vi "古田户外一体站流程平行样自动启动.vi"(9 "参数":T1={"是否启用仪器"=FALSE, "CODMn"={"启动测量模式"={"测量模式"=enum."水样测量"}, "确定按钮"=TRUE}, "启动模块"={"氨氮1"=FALSE, "总磷1"=FALSE, " COD1"=FALSE}, "常规启动"=FALSE, "直接启动"=FALSE}) -> ()   [LabVIEW 2016, in "质控单元.lvlib"]
uses:
  PLC/PLC.lvlib
panel:
  out "COD平行样测完标志":bool
  out "氨氮总磷平行样测完标志":bool
  out "枚举 2":enum16{"初始化", "采配水启动", "等待", "配水", "排水", "结束"}(ring)
  out "枚举":enum16{"初始化", "采配水启动", "等待", "配水", "排水", "结束"}(ring)
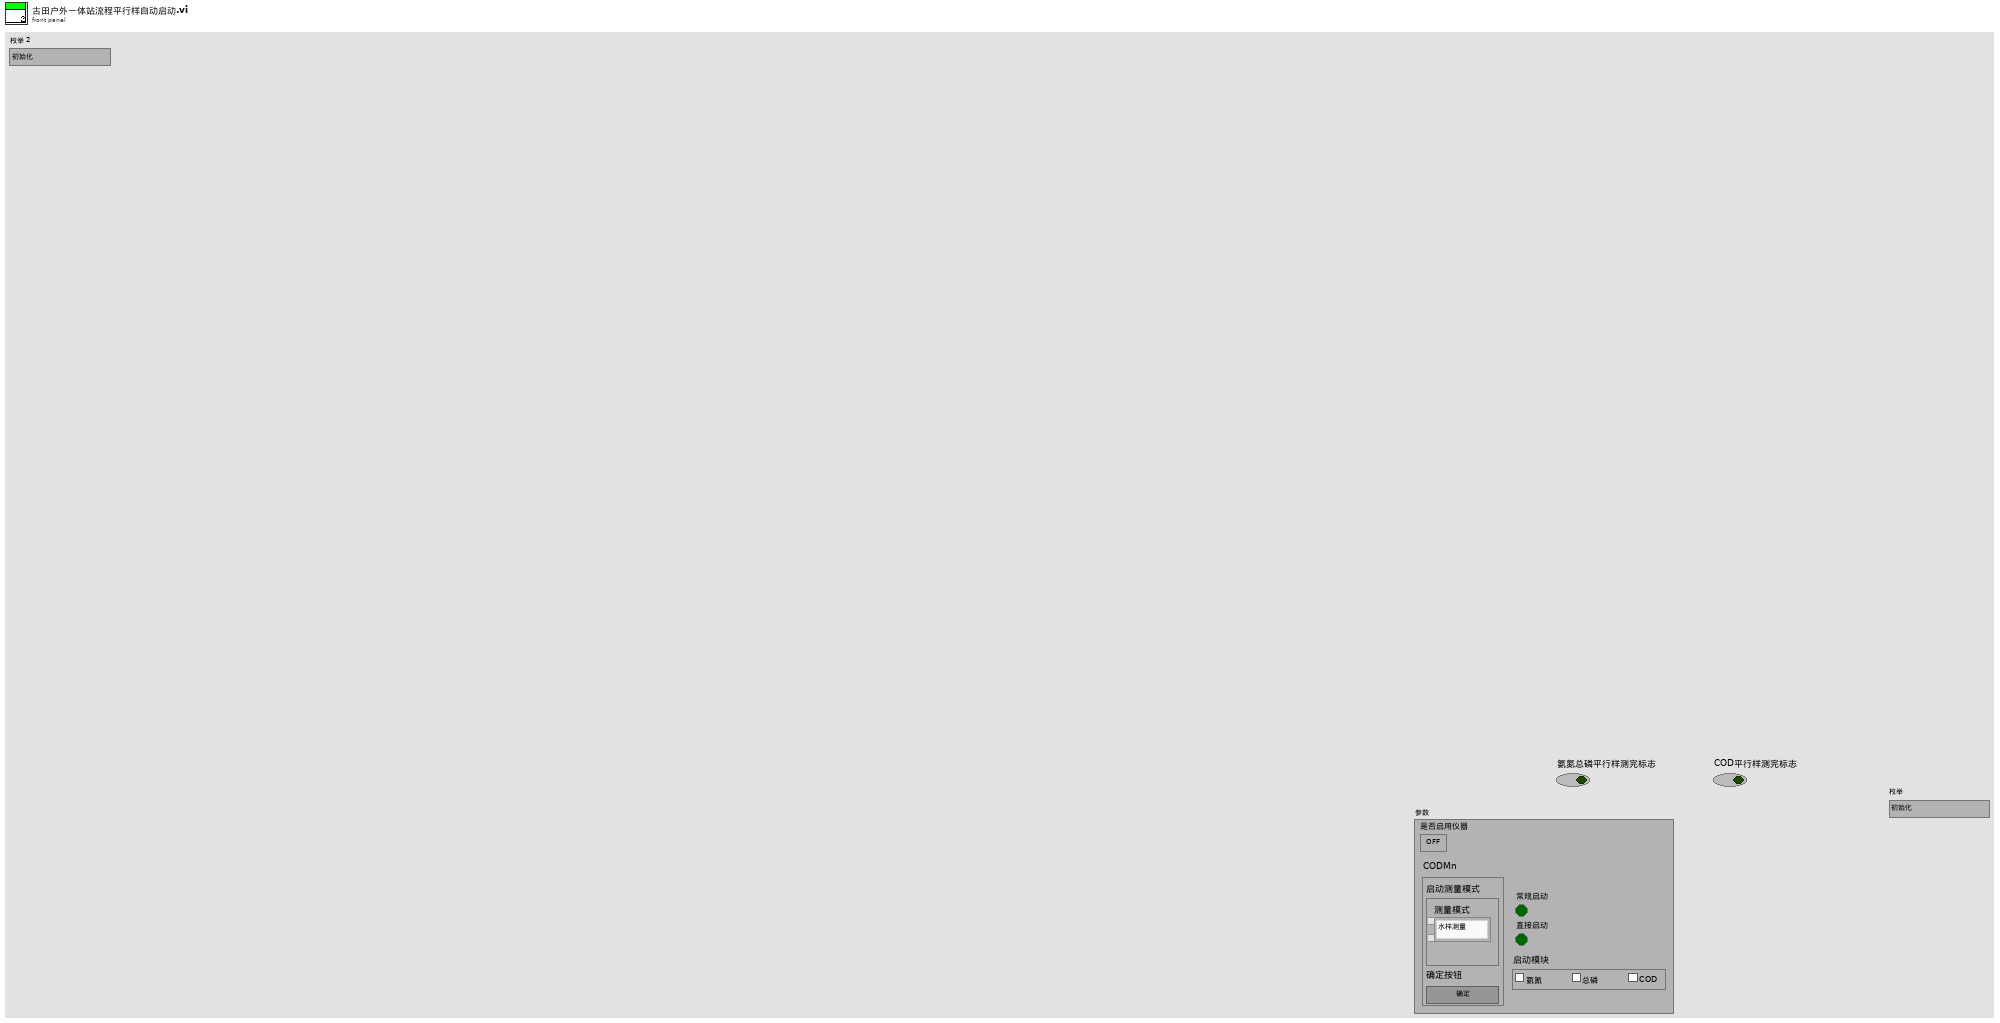
[diagram p1: front panel]
types:
  T1 = cluster{"是否启用仪器":bool, "CODMn":cluster{"启动测量模式":cluster{"测量模式":enum16{"水样测量", "标样核查", "加标回收", "平行样", "校零", "校标"}}, "确定按钮":bool}, "启动模块":cluster{"氨氮1":bool, "总磷1":bool, " COD1":bool}, "常规启动":bool, "直接启动":bool}
  T2 = cluster{"命令":string, cluster{"starting address":u16, "holding register value":u16}}
  T3 = cluster{"R0":i16, "R1":i16, "R2":i16, "R3":i16, "R4":i16, "R5":i16, "R6":i16, "R7":i16, "R8":i16, "R9":i16, "R10":i16, "R11":i16, "R12":i16, "R13":i16, "R14":i16, "R15":i16, "R16":i16, "R17":i16, "R18":i16, "R19":i16}
  T4 = enum32{"Bad", "Idle", "Run top level", "Running"}
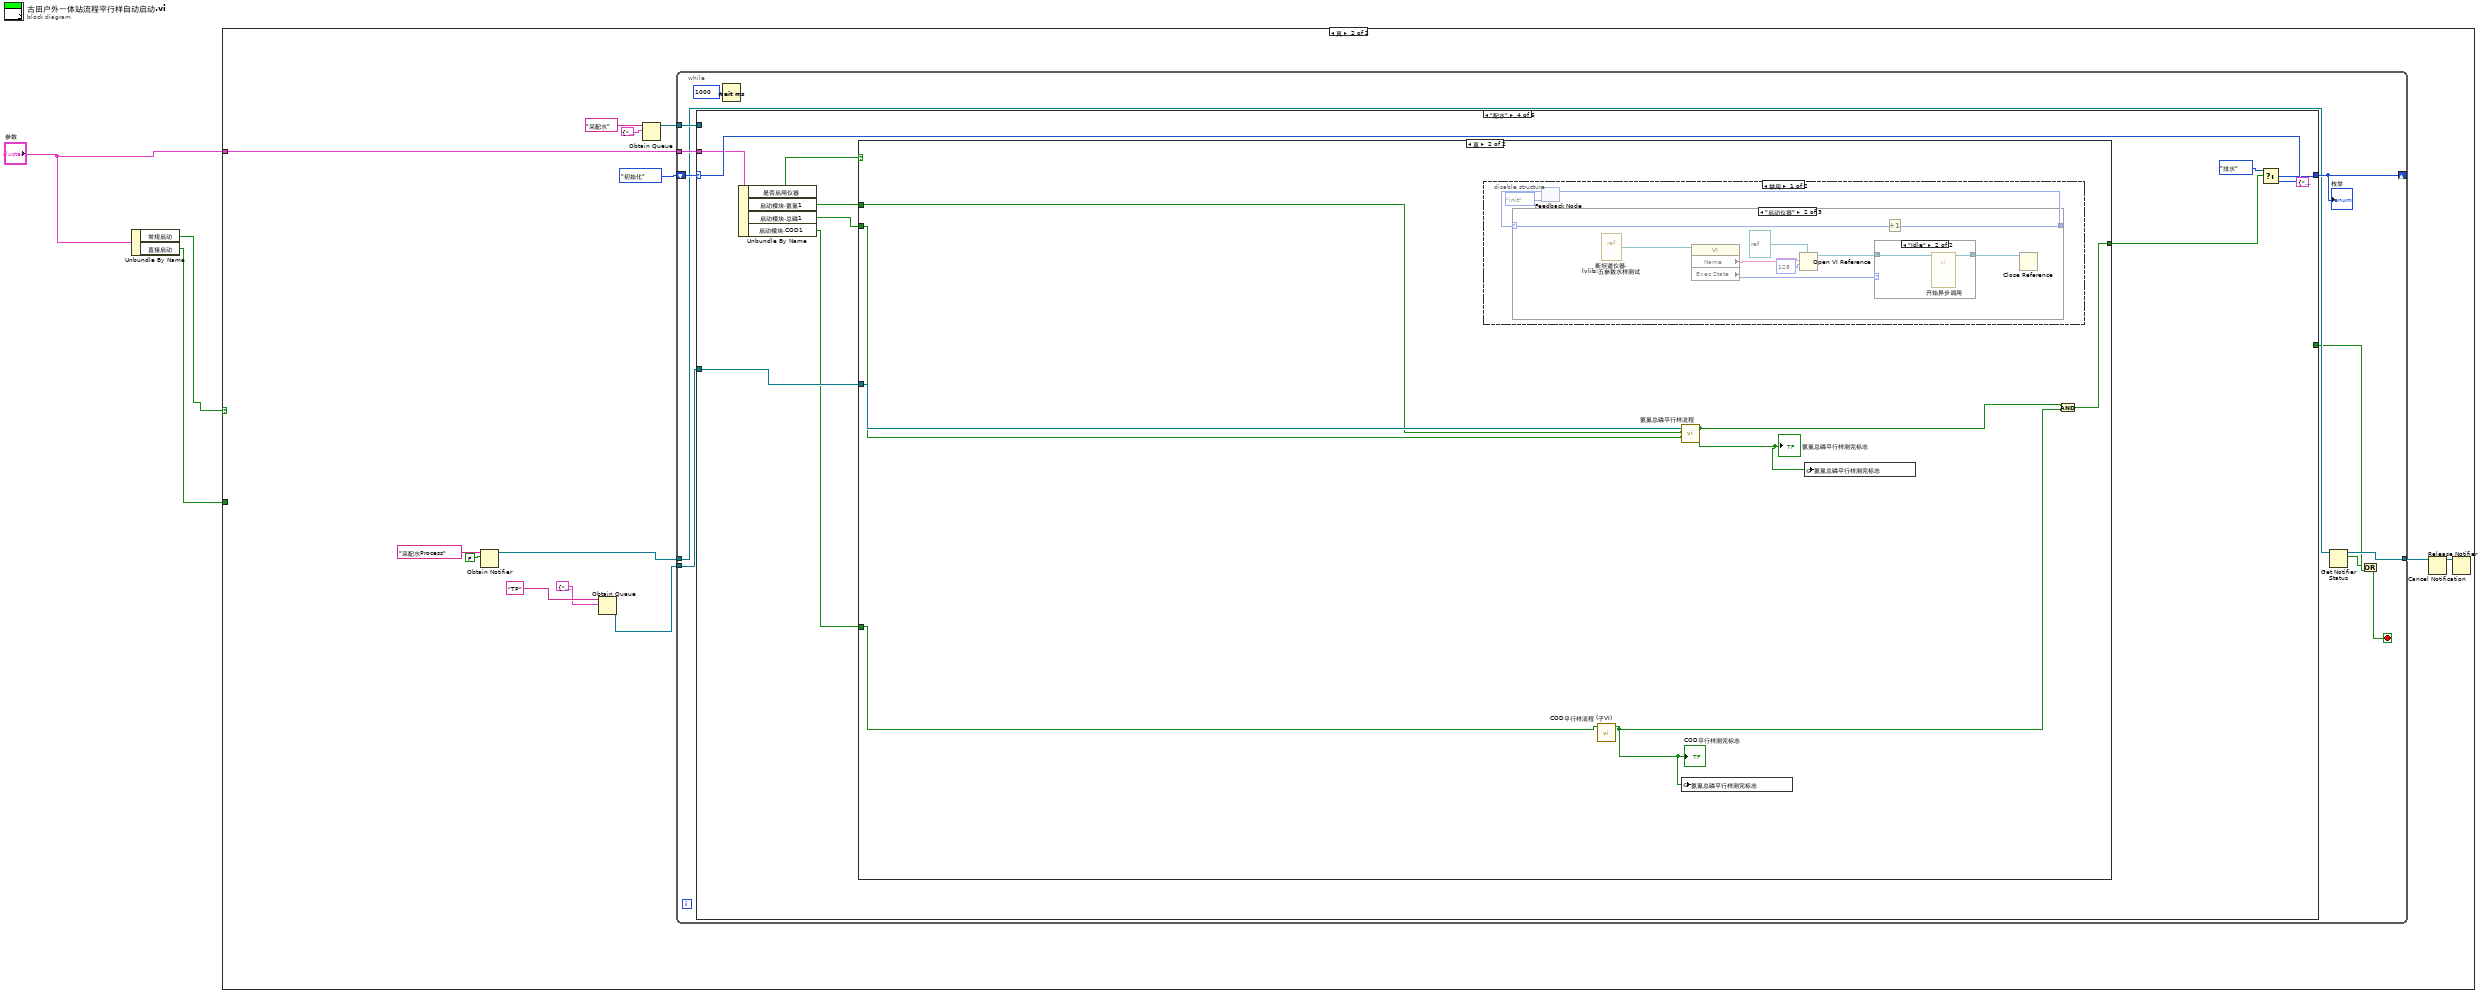
[diagram p0: block diagram]
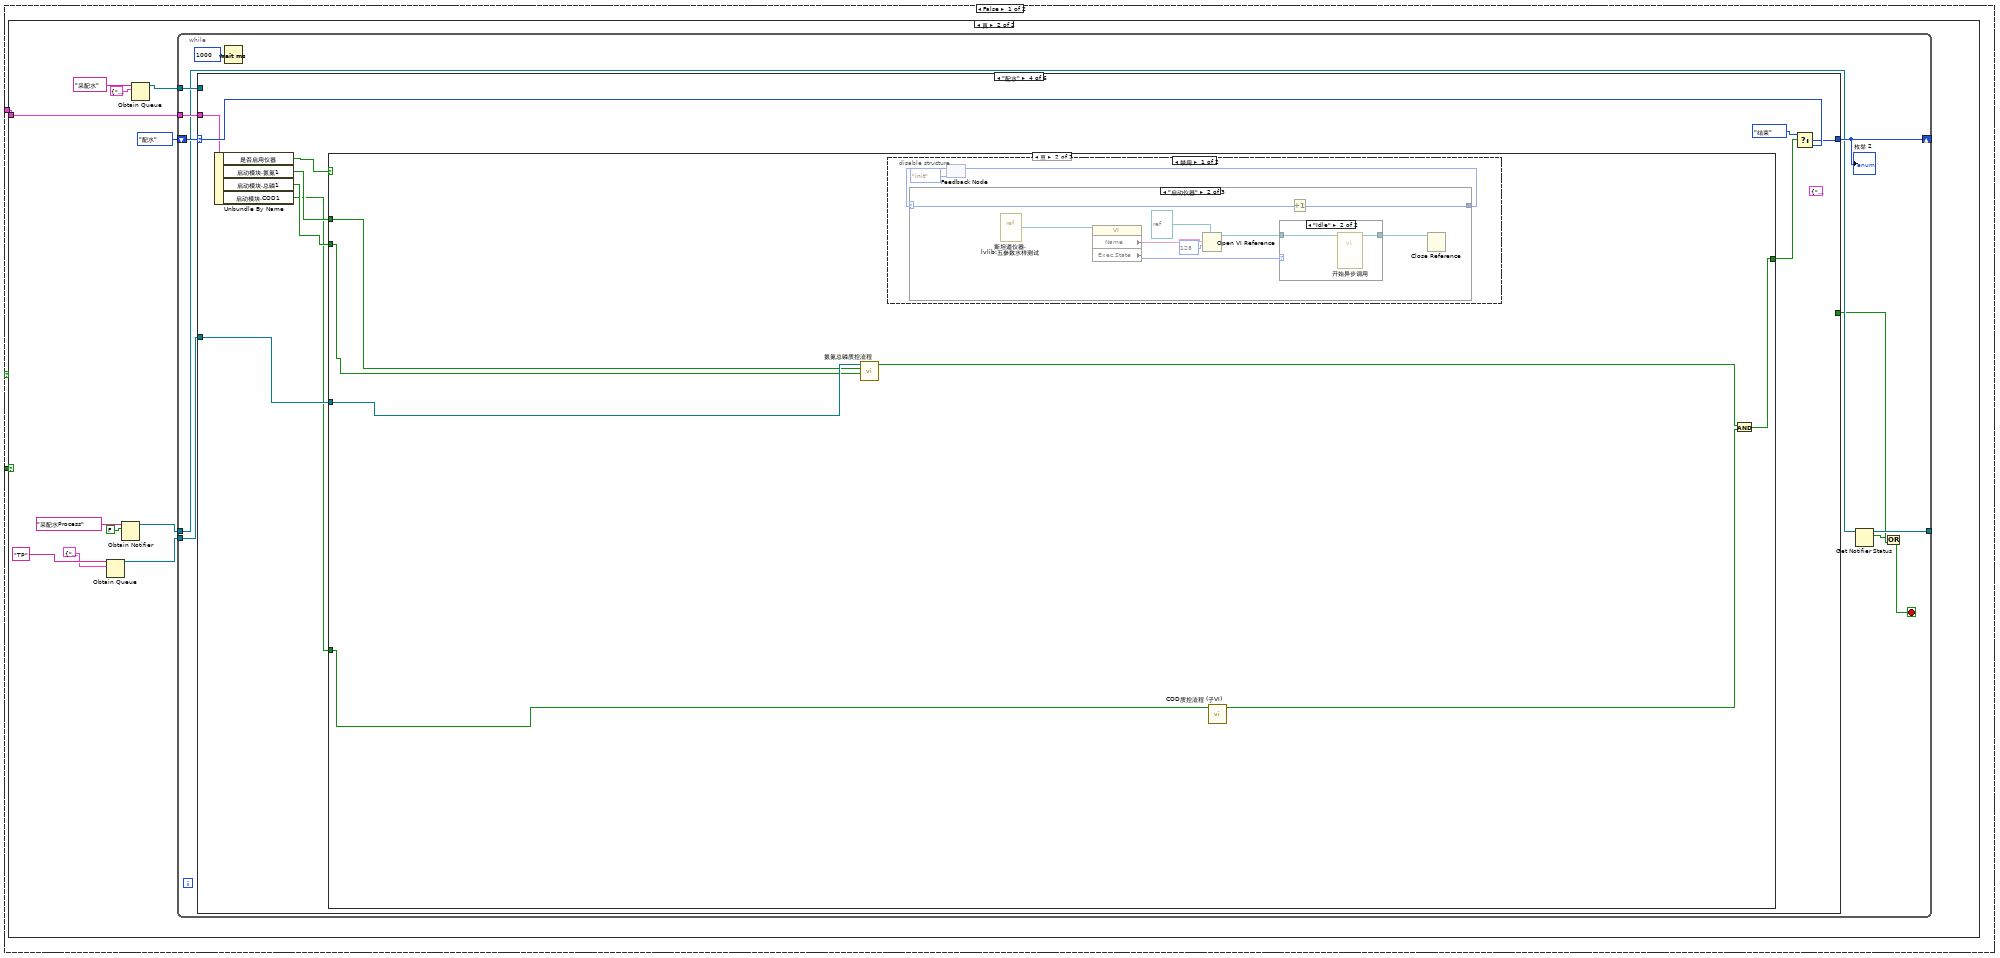
[diagram p2: hidden frame]
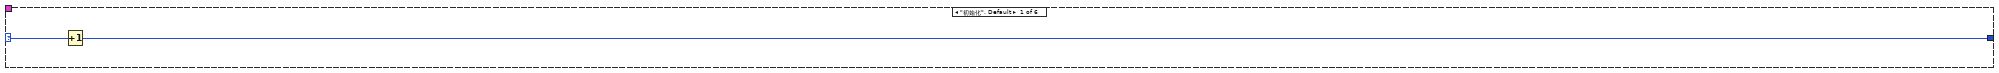
[diagram p4: hidden frame]
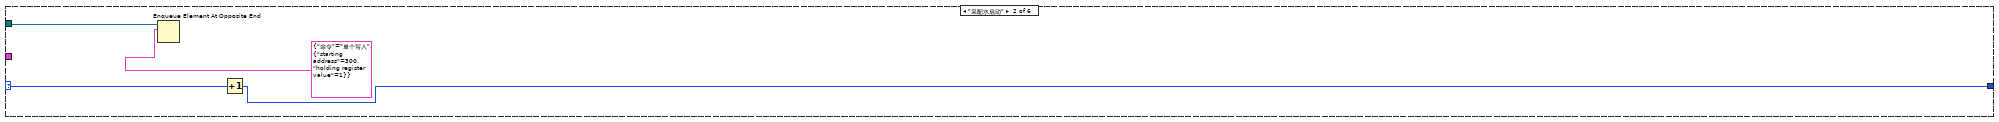
[diagram p5: hidden frame]
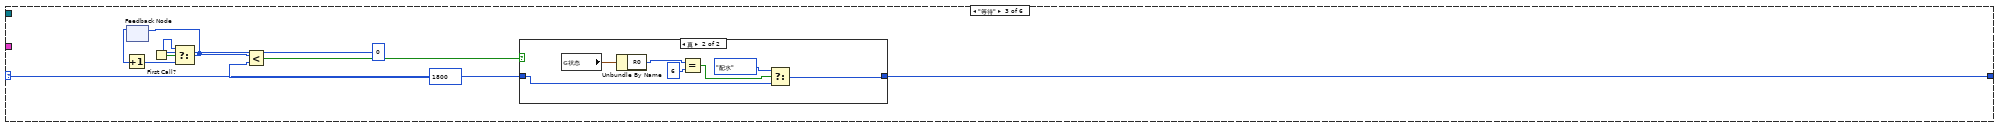
[diagram p6: hidden frame]
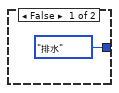
[diagram p7: hidden frame]
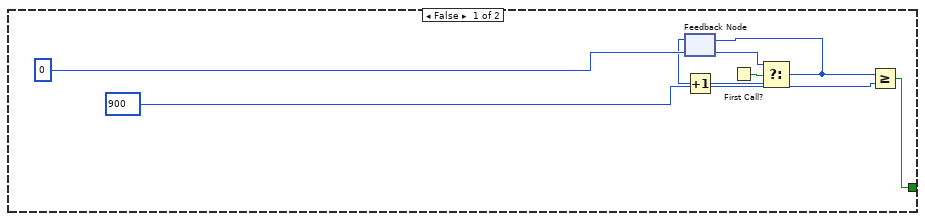
[diagram p8: hidden frame]
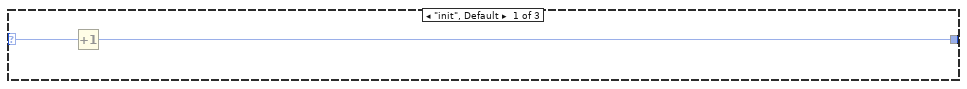
[diagram p9: hidden frame]
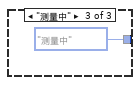
[diagram p11: hidden frame]
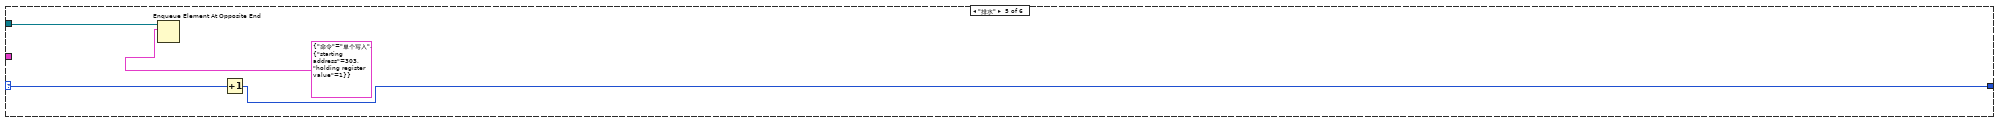
[diagram p13: hidden frame]
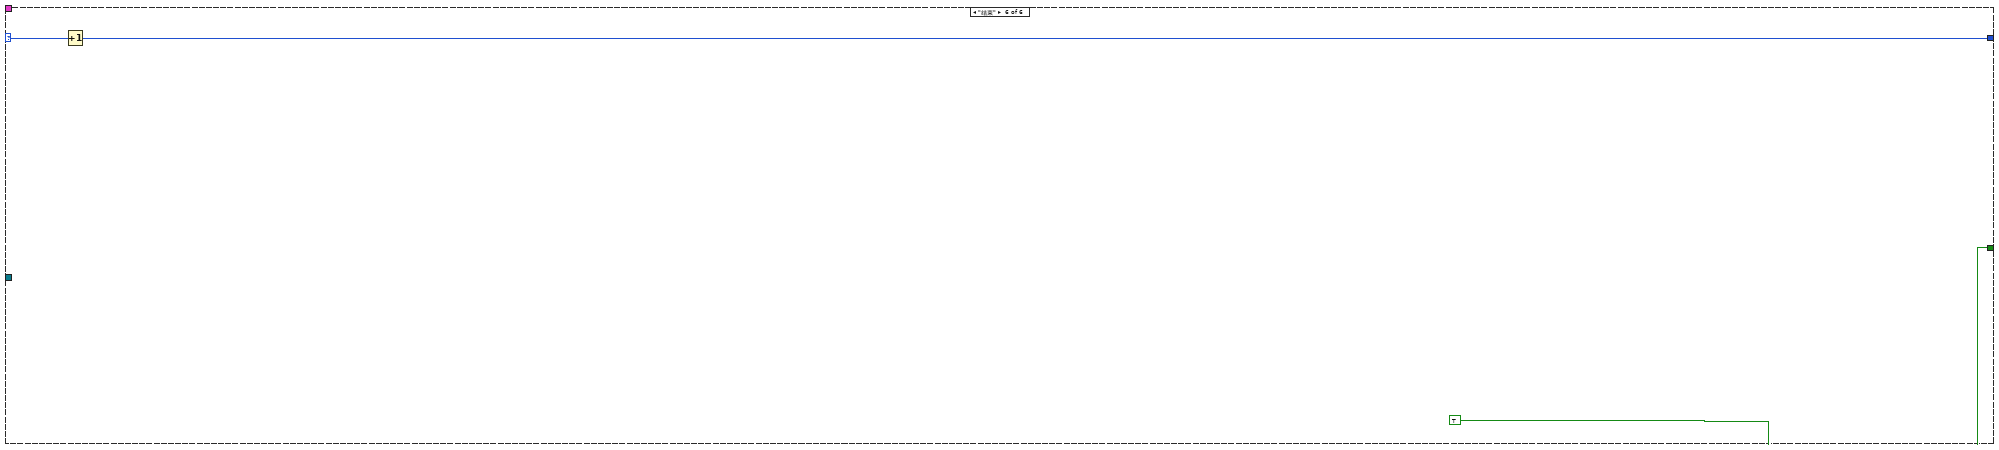
[diagram p14: hidden frame]
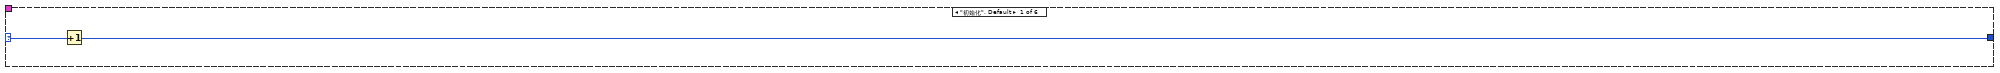
[diagram p15: hidden frame]
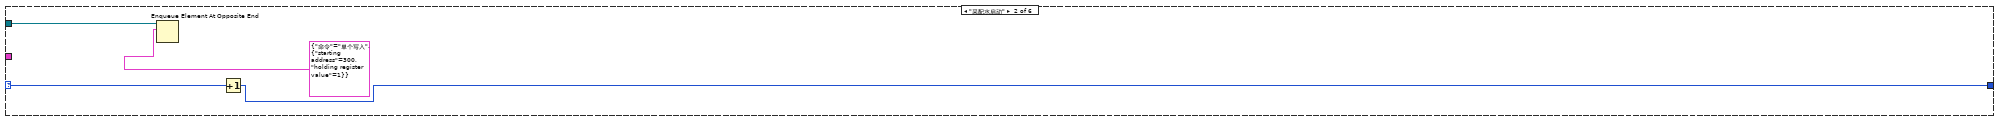
[diagram p16: hidden frame]
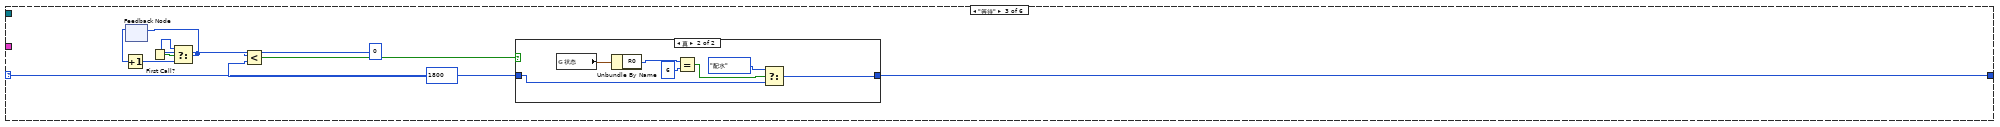
[diagram p17: hidden frame]
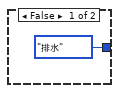
[diagram p18: hidden frame]
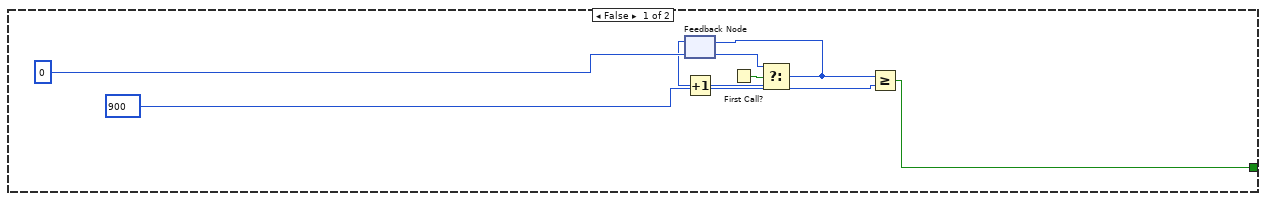
[diagram p19: hidden frame]
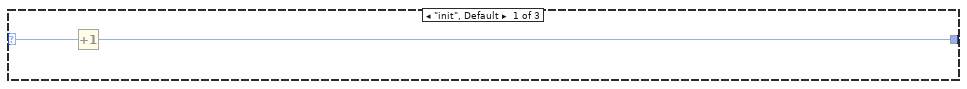
[diagram p20: hidden frame]
diagram:
  n1 = Unbundle By Name("参数") -> ("常规启动"=w2:bool, "直接启动"=w1:bool)
  n2 = case shown="真" w2 {
    tunnel: "参数" -> [w4 w100]
    tunnel: w1 -> [w5 _]
    frame False {
      n3 = case shown="真" w5 {
        tunnel: w4 -> [_ w15]
        frame False {
        }
        frame True {
          n4 = Obtain Queue(name (unnamed)="TP" ("名称（未命名）"), element data type=cluster{"命令":string, "data":variant} {"命令"="", "data"=variant}) -> (queue out=w6:refnum<queue>)  [unwired: 3 in, 2 out]
          n5 = Obtain Notifier(name (unnamed)="采配水Process" ("名称（未命名）"), notification data type=FALSE) -> (notifier out=w9:refnum<notifier>)  [unwired: 2 in, 2 out]
          n6 = Obtain Queue(name (unnamed)="采配水" ("名称（未命名）"), element data type=cluster{"命令":string, "数据":variant} {"命令"="", "数据"=variant}) -> (queue out=w12:refnum<queue>)  [unwired: 3 in, 2 out]
          n7 = while {
            tunnel: w12 -> [w27]
            shift-right: [w25] -> _
            shift-left: enum16{"初始化", "采配水启动", "等待", "配水", "排水", "结束"}."配水" ("枚举") -> [w26]
            tunnel: w6 -> [w23]
            tunnel: w15 -> [w22]
            tunnel: w9 -> [w21]
            tunnel: [w20] -> _
            stop <- w19 stop-if-true
            n8 = case shown="\"配水\"" w26 {
              selector: w26 -> [w29 w31 w40 w59 w94 w99]
              tunnel: w27 -> [_ w32 _ _ w95 _]
              tunnel: [w28 w30 w39 w58 w93 w98] -> w25
              tunnel: [_ _ _ _ _ TRUE] -> w18
              tunnel: w23 -> [_ _ _ w57 _ _]
              tunnel: w22 -> [_ _ _ w54 _ _]
              frame "初始化", Default {
                n9 = Increment(x=w29) -> (x+1=w28:enum16{"初始化", "采配水启动", "等待", "配水", "排水", "结束"})
              }
              frame "采配水启动" {
                n10 = Enqueue Element At Opposite End(queue=w32, element=T2 {"命令"="单个写入", {"starting address"=300, "holding register value"=1}} ("元素")) -> ()  [unwired: 2 in, 3 out]
                n11 = Increment(x=w31) -> (x+1=w30:enum16{"初始化", "采配水启动", "等待", "配水", "排水", "结束"})
              }
              frame "等待" {
                n12 = feedback #1() -> (w36:i32)  [unwired: 1 in]
                n13 = Increment(x=w36) -> (x+1=w35:i32)
                n14 = First Call?() -> (First Call?: T/F=w37:bool)
                n15 = Select(t=0, s=w37, f=w35) -> (s? t:f=w34:i32)
                n16 = feedback-in #1(w34) -> ()
                n17 = Less?(x=w34, y=1800) -> (x < y?=w41:bool)
                n18 = case shown="真" w41 {
                  tunnel: w40 -> [_ w45]
                  tunnel: [enum16{"初始化", "采配水启动", "等待", "配水", "排水", "结束"}."排水" ("枚举") w44] -> w39
                  frame False {
                  }
                  frame True {
                    n19 = global read "采配水全局变量.vi" "状态"() -> (w50:T3)
                    n20 = Unbundle By Name(w50) -> ("R0"=w49:i16)
                    n21 = Equal?(x=w49, y=i16 6) -> (x = y?=w47:bool)
                    n22 = Select(t=enum16{"初始化", "采配水启动", "等待", "配水", "排水", "结束"}."配水" ("枚举"), s=w47, f=w45) -> (s? t:f=w44:enum16{"初始化", "采配水启动", "等待", "配水", "排水", "结束"})
                  }
                }
              }
              frame "配水" {
                (unwired) cluster{"命令":string, "data":variant} {"命令"="启动", "data"=variant(cluster{"站号":u16, "控制命令输出":u16[]} {"站号"=1, "控制命令输出"=[256, 0]})} ("元素")
                n23 = Unbundle By Name(w54) -> ("是否启用仪器"=w56:bool, "启动模块.氨氮1"=w52:bool, "启动模块.总磷1"=w53:bool, "启动模块.COD1"=w51:bool)
                n24 = case shown="真" w56 {
                  tunnel: w57 -> [_ w73]
                  tunnel: [w61 w74] -> w55
                  tunnel: w53 -> [_ w70]
                  tunnel: w52 -> [_ w71]
                  tunnel: w51 -> [_ w69]
                  frame False {
                    n25 = feedback #2() -> (w65:i32)  [unwired: 1 in]
                    n26 = Increment(x=w65) -> (x+1=w64:i32)
                    n27 = First Call?() -> (First Call?: T/F=w66:bool)
                    n28 = Select(t=0, s=w66, f=w64) -> (s? t:f=w62:i32)
                    n29 = feedback-in #2(w62) -> ()
                    n30 = Greater Or Equal?(x=w62, y=900) -> (x >= y?=w61:bool)
                  }
                  frame True {
                    n31 = call "氨氮总磷质控流程.vi"("总磷1"=w70, "氨氮1"=w71, "队列输入"=w73) -> ("布尔"=w72:bool)  [unwired: 8 in]
                    n32 = disable-structure shown="禁用" {
                      frame Disabled {
                        n33 = feedback #3(enum16{"init", "启动仪器", "测量中"}."init") -> (w76:enum16{"init", "启动仪器", "测量中"})
                        n34 = case shown="\"启动仪器\"" w76 {
                          selector: w76 -> [w79 w88 _]
                          tunnel: [w78 w87 enum16{"init", "启动仪器", "测量中"}."测量中"] -> w77
                          frame "init", Default {
                            n35 = Increment(x=w79) -> (x+1=w78:enum16{"init", "启动仪器", "测量中"})
                          }
                          frame "启动仪器" {
                            n36 = vi-ref "斯坦道仪器.lvlib:五参数水样测试.vi"() -> (w80:refnum<vi>)
                            n37 = property class="VI"(reference=w80) -> ("Name"=w84:string, "Exec.State"=w82:T4)  [unwired: 1 in, 2 out]
                            n38 = Open VI Reference(type specifier VI Refnum (for type only)=refnum<vi> refnum ("类型说明符VI引用句柄（仅用于类型）"), vi path=w84, options=128 ("选项")) -> (vi reference=w83:refnum<vi>)  [unwired: 3 in, 1 out]
                            n39 = case shown="\"Idle\"" w82 {
                              tunnel: w83 -> [w89 w91]
                              tunnel: [w89 w90] -> w81
                              frame "Bad", Default {
                              }
                              frame "Idle" {
                                n40 = call-by-ref "开始异步调用"(reference=w91) -> (reference out=w90:refnum<vi>)  [unwired: 13 in, 1 out]
                              }
                            }
                            n41 = Increment(x=w88) -> (x+1=w87:enum16{"init", "启动仪器", "测量中"})
                            n42 = Close Reference(reference=w81) -> ()  [unwired: 1 in, 1 out]
                          }
                          frame "测量中" {
                          }
                        }
                        n43 = feedback-in #3(w77) -> ()
                      }
                      frame Enabled {
                      }
                    }
                    n44 = call "COD质控流程 (子VI).vi"("COD1"=w69) -> ("布尔"=w68:bool)  [unwired: 10 in]
                    n45 = And(x=w72, y=w68) -> (x .and. y?=w74:bool)
                  }
                }
                n46 = Select(t=enum16{"初始化", "采配水启动", "等待", "配水", "排水", "结束"}."结束" ("枚举"), s=w55, f=w59) -> (s? t:f=w58:enum16{"初始化", "采配水启动", "等待", "配水", "排水", "结束"})
              }
              frame "排水" {
                n47 = Enqueue Element At Opposite End(queue=w95, element=T2 {"命令"="单个写入", {"starting address"=303, "holding register value"=1}} ("元素")) -> ()  [unwired: 2 in, 3 out]
                n48 = Increment(x=w94) -> (x+1=w93:enum16{"初始化", "采配水启动", "等待", "配水", "排水", "结束"})
              }
              frame "结束" {
                n49 = Increment(x=w99) -> (x+1=w98:enum16{"初始化", "采配水启动", "等待", "配水", "排水", "结束"})
              }
            }
            "枚举 2" <- w25
            n50 = Wait (ms)(milliseconds to wait=u32 1000 ("等待时间（毫秒）")) -> ()  [unwired: 1 out]
            n51 = Get Notifier Status(notifier=w21) -> (notifier out=w20:refnum<notifier>, current notification=w17:bool)  [unwired: 1 in, 3 out]
            n52 = Or(x=w17, y=w18) -> (x .or. y?=w19:bool)
          }
        }
      }
    }
    frame True {
      n53 = Obtain Notifier(name (unnamed)="采配水Process" ("名称（未命名）"), notification data type=FALSE) -> (notifier out=w103:refnum<notifier>)  [unwired: 2 in, 2 out]
      n54 = Obtain Queue(name (unnamed)="TP" ("名称（未命名）"), element data type=cluster{"命令":string, "data":variant} {"命令"="", "data"=variant}) -> (queue out=w106:refnum<queue>)  [unwired: 3 in, 2 out]
      n55 = Obtain Queue(name (unnamed)="采配水" ("名称（未命名）"), element data type=cluster{"命令":string, "数据":variant} {"命令"="", "数据"=variant}) -> (queue out=w110:refnum<queue>)  [unwired: 3 in, 2 out]
      n56 = while {
        tunnel: w110 -> [w123]
        shift-right: [w121] -> _
        shift-left: enum16{"初始化", "采配水启动", "等待", "配水", "排水", "结束"}."初始化" ("枚举") -> [w122]
        tunnel: w106 -> [w119]
        tunnel: w100 -> [w118]
        tunnel: w103 -> [w117]
        tunnel: [w116] -> w102
        stop <- w115 stop-if-true
        n57 = case shown="\"配水\"" w122 {
          selector: w122 -> [w125 w127 w136 w155 w190 w195]
          tunnel: w123 -> [_ w128 _ _ w191 _]
          tunnel: [w124 w126 w135 w154 w189 w194] -> w121
          tunnel: [_ _ _ _ _ TRUE] -> w114
          tunnel: w119 -> [_ _ _ w153 _ _]
          tunnel: w118 -> [_ _ _ w150 _ _]
          frame "初始化", Default {
            n58 = Increment(x=w125) -> (x+1=w124:enum16{"初始化", "采配水启动", "等待", "配水", "排水", "结束"})
          }
          frame "采配水启动" {
            n59 = Enqueue Element At Opposite End(queue=w128, element=T2 {"命令"="单个写入", {"starting address"=300, "holding register value"=1}} ("元素")) -> ()  [unwired: 2 in, 3 out]
            n60 = Increment(x=w127) -> (x+1=w126:enum16{"初始化", "采配水启动", "等待", "配水", "排水", "结束"})
          }
          frame "等待" {
            n61 = feedback #4() -> (w132:i32)  [unwired: 1 in]
            n62 = Increment(x=w132) -> (x+1=w131:i32)
            n63 = First Call?() -> (First Call?: T/F=w133:bool)
            n64 = Select(t=0, s=w133, f=w131) -> (s? t:f=w130:i32)
            n65 = feedback-in #4(w130) -> ()
            n66 = Less?(x=w130, y=1800) -> (x < y?=w137:bool)
            n67 = case shown="真" w137 {
              tunnel: w136 -> [_ w141]
              tunnel: [enum16{"初始化", "采配水启动", "等待", "配水", "排水", "结束"}."排水" ("枚举") w140] -> w135
              frame False {
              }
              frame True {
                n68 = global read "采配水全局变量.vi" "状态"() -> (w146:T3)
                n69 = Unbundle By Name(w146) -> ("R0"=w145:i16)
                n70 = Equal?(x=w145, y=i16 6) -> (x = y?=w143:bool)
                n71 = Select(t=enum16{"初始化", "采配水启动", "等待", "配水", "排水", "结束"}."配水" ("枚举"), s=w143, f=w141) -> (s? t:f=w140:enum16{"初始化", "采配水启动", "等待", "配水", "排水", "结束"})
              }
            }
          }
          frame "配水" {
            (unwired) cluster{"命令":string, "data":variant} {"命令"="启动", "data"=variant(cluster{"站号":u16, "控制命令输出":u16[]} {"站号"=1, "控制命令输出"=[256, 0]})} ("元素")
            n72 = Unbundle By Name(w150) -> ("是否启用仪器"=w152:bool, "启动模块.氨氮1"=w148:bool, "启动模块.总磷1"=w149:bool, "启动模块.COD1"=w147:bool)
            n73 = case shown="真" w152 {
              tunnel: w153 -> [_ w170]
              tunnel: [w157 w167] -> w151
              tunnel: w149 -> [_ w168]
              tunnel: w148 -> [_ w169]
              tunnel: w147 -> [_ w166]
              frame False {
                n74 = feedback #5() -> (w161:i32)  [unwired: 1 in]
                n75 = Increment(x=w161) -> (x+1=w160:i32)
                n76 = First Call?() -> (First Call?: T/F=w162:bool)
                n77 = Select(t=0, s=w162, f=w160) -> (s? t:f=w158:i32)
                n78 = feedback-in #5(w158) -> ()
                n79 = Greater Or Equal?(x=w158, y=900) -> (x >= y?=w157:bool)
              }
              frame True {
                n80 = disable-structure shown="禁用" {
                  frame Disabled {
                    n81 = feedback #6(enum16{"init", "启动仪器", "测量中"}."init") -> (w172:enum16{"init", "启动仪器", "测量中"})
                    n82 = case shown="\"启动仪器\"" w172 {
                      selector: w172 -> [w175 w184 _]
                      tunnel: [w174 w183 enum16{"init", "启动仪器", "测量中"}."测量中"] -> w173
                      frame "init", Default {
                        n83 = Increment(x=w175) -> (x+1=w174:enum16{"init", "启动仪器", "测量中"})
                      }
                      frame "启动仪器" {
                        n84 = vi-ref "斯坦道仪器.lvlib:五参数水样测试.vi"() -> (w176:refnum<vi>)
                        n85 = property class="VI"(reference=w176) -> ("Name"=w180:string, "Exec.State"=w178:T4)  [unwired: 1 in, 2 out]
                        n86 = Open VI Reference(type specifier VI Refnum (for type only)=refnum<vi> refnum ("类型说明符VI引用句柄（仅用于类型）"), vi path=w180, options=128 ("选项")) -> (vi reference=w179:refnum<vi>)  [unwired: 3 in, 1 out]
                        n87 = case shown="\"Idle\"" w178 {
                          tunnel: w179 -> [w185 w187]
                          tunnel: [w185 w186] -> w177
                          frame "Bad", Default {
                          }
                          frame "Idle" {
                            n88 = call-by-ref "开始异步调用"(reference=w187) -> (reference out=w186:refnum<vi>)  [unwired: 13 in, 1 out]
                          }
                        }
                        n89 = Increment(x=w184) -> (x+1=w183:enum16{"init", "启动仪器", "测量中"})
                        n90 = Close Reference(reference=w177) -> ()  [unwired: 1 in, 1 out]
                      }
                      frame "测量中" {
                      }
                    }
                    n91 = feedback-in #6(w173) -> ()
                  }
                  frame Enabled {
                  }
                }
                n92 = call "COD平行样流程 (子VI).vi"("COD1"=w166) -> ("布尔"=w164:bool)  [unwired: 10 in]
                "COD平行样测完标志" <- w164
                n93 = call "氨氮总磷平行样流程.vi"("总磷1"=w168, "氨氮1"=w169, "队列输入"=w170) -> ("布尔"=w165:bool)  [unwired: 8 in]
                "氨氮总磷平行样测完标志" <- w165
                n94 = global write "质控测完标志全局 1.vi" "氨氮总磷平行样测完标志"(w164) -> ()
                n95 = global write "质控测完标志全局 1.vi" "氨氮总磷平行样测完标志"(w165) -> ()
                n96 = And(x=w165, y=w164) -> (x .and. y?=w167:bool)
              }
            }
            n97 = Select(t=enum16{"初始化", "采配水启动", "等待", "配水", "排水", "结束"}."排水" ("枚举"), s=w151, f=w155) -> (s? t:f=w154:enum16{"初始化", "采配水启动", "等待", "配水", "排水", "结束"})
          }
          frame "排水" {
            n98 = Enqueue Element At Opposite End(queue=w191, element=T2 {"命令"="单个写入", {"starting address"=303, "holding register value"=1}} ("元素")) -> ()  [unwired: 2 in, 3 out]
            n99 = Increment(x=w190) -> (x+1=w189:enum16{"初始化", "采配水启动", "等待", "配水", "排水", "结束"})
          }
          frame "结束" {
            n100 = Increment(x=w195) -> (x+1=w194:enum16{"初始化", "采配水启动", "等待", "配水", "排水", "结束"})
          }
        }
        "枚举" <- w121
        n101 = Wait (ms)(milliseconds to wait=u32 1000 ("等待时间（毫秒）")) -> ()  [unwired: 1 out]
        n102 = Get Notifier Status(notifier=w117) -> (notifier out=w116:refnum<notifier>, current notification=w113:bool)  [unwired: 1 in, 3 out]
        n103 = Or(x=w113, y=w114) -> (x .or. y?=w115:bool)
      }
      n104 = Cancel Notification(0:w102) -> (8:w101:refnum<notifier>)  [unwired: 1 in, 2 out]
      n105 = Release Notifier(notifier=w101) -> ()  [unwired: 2 in, 3 out]
    }
  }
